vi "ser.bools.vi"(11 "orderbook.command":T1) -> (3 "Numeric":u32 format="%.0x")   [LabVIEW 2020, in "fpganow.common.fpga.lvlib"]
uses:
  fpganow.common.fpga.lvlib
  orderbook.command.ctl
  orderbook.command.type.ctl
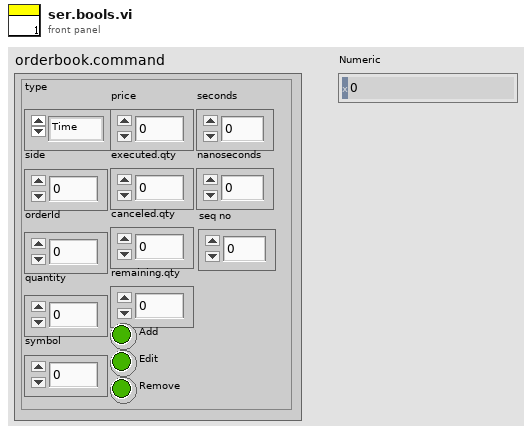
[diagram p1: front panel]
types:
  T1 = typedef "fpganow.common.fpga.lvlib/orderbook.command.ctl" = cluster{"type":T2, "side":u8, "orderId ":u64, "quantity":u32, "symbol":u64, "price":u64, "executed.qty":u32, "canceled.qty":u32, "remaining.qty":u32, "seconds":u64, "nanoseconds":u64, "Add":bool, "Edit":bool, "Remove":bool, "seq no":u32}
  T2 = typedef "fpganow.common.fpga.lvlib/orderbook.command.type.ctl" = enum8{"Time", "AddOrder", "OrderExecuted", "OrderExecutedAtPrice", "ReduceSize", "ModifyOrder", "DeleteOrder", "Get.Everything", "Get.All.Orders", "Get.Top"}
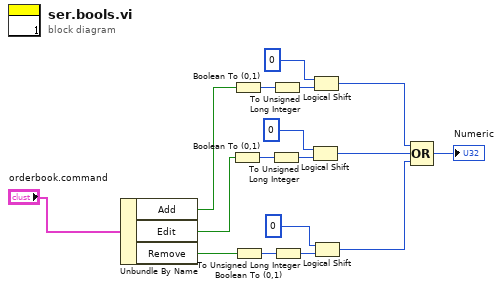
[diagram p0: block diagram]
diagram:
  n1 = Unbundle By Name("orderbook.command") -> ("Add"=w12:bool, "Edit"=w6:bool, "Remove"=w1:bool)
  n2 = Boolean To (0,1)(Boolean=w6) -> (0, 1=w9:i16)
  n3 = Boolean To (0,1)(Boolean=w12) -> (0, 1=w13:i16)
  n4 = Boolean To (0,1)(Boolean=w1) -> (0, 1=w5:i16)
  n5 = To Unsigned Long Integer(number=w9) -> (unsigned 32bit integer=w8:u32)
  n6 = To Unsigned Long Integer(number=w13) -> (unsigned 32bit integer=w11:u32)
  n7 = To Unsigned Long Integer(number=w5) -> (unsigned 32bit integer=w4:u32)
  n8 = Logical Shift(y=u32 0, x=w8) -> (x << y=w7:u32)
  n9 = Logical Shift(y=u32 0, x=w11) -> (x << y=w15:u32)
  n10 = Logical Shift(y=u32 0, x=w4) -> (x << y=w3:u32)
  n11 = Compound Arithmetic op=OR(w15, w7, w3) -> (→"Numeric":u32)
